vi "Write Visible_.vi"(8 "error in (no error)":errorcluster, 10 "Visible?":bool, 11 "Visible Assertion in":refnum<class "Visible Assertion.lvclass">) -> (0 "error out":errorcluster, 3 "Visible Assertion out":refnum<class "Visible Assertion.lvclass">)   [LabVIEW 2020, in "MacroAssert.lvlib" / "Visible Assertion.lvclass"]
uses:
  Visible Assertion.lvclass
  Visible Assertion.lvclass/Visible Assertion.ctl
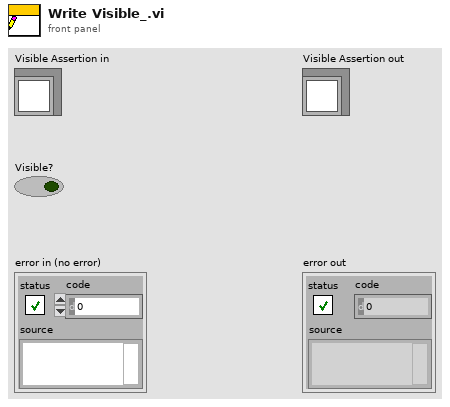
[diagram p1: front panel]
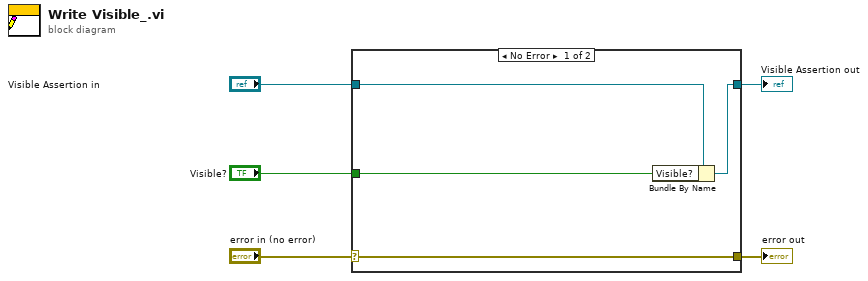
[diagram p0: block diagram]
diagram:
  n1 = case shown="No Error" "error in (no error)" {
    selector: "error in (no error)" -> [w9 w10]
    tunnel: [w9 w10] -> w4
    tunnel: [w7 w11] -> w2
    tunnel: "Visible Assertion in" -> [w8 w11]
    tunnel: "Visible?" -> [w6 _]
    frame No Error {
      n2 = Bundle By Name(cluster=w8, "Visible?"=w6) -> (w7:refnum<class "Visible Assertion.lvclass">)
    }
    frame Error {
    }
  }
  "error out" <- w4
  "Visible Assertion out" <- w2
